vi "Test Sweep API.vi"   [LabVIEW 2019]
uses:
  c3f68086-2c71-4676-baf4-799858c1ae09.vi
  1559a243-b7fb-4211-921b-e5aebecb1ff1.vi
  <vilib>/Analysis/NI_AALBase.lvlib
  <vilib>/Analysis/1siggen.llb/Ramp Pattern by Samples.vi
  cdfe988a-f24c-4ea6-9edf-21cd4fa2a456.vi
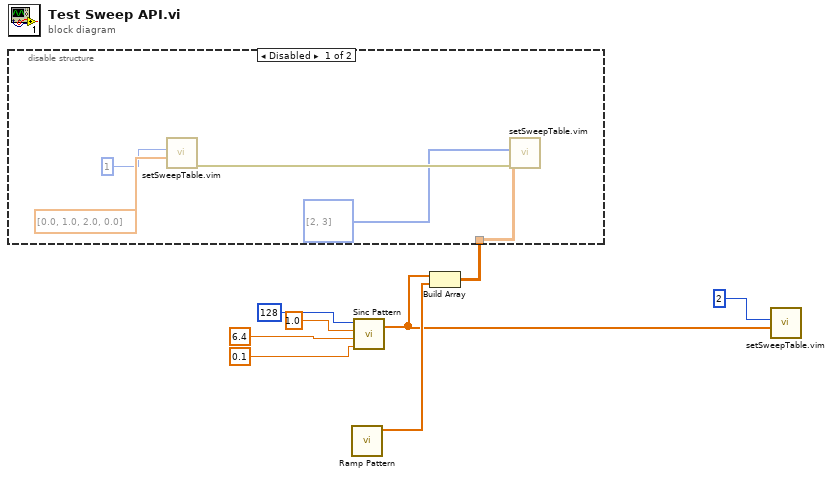
[diagram p0: block diagram]
diagram:
  n1 = call-poly <vilib>:"Ramp Pattern.vi"() -> ("Ramp Pattern"=w7:dbl[])  [unwired: 10 in, 1 out]
  n2 = call <vilib>:"Sinc Pattern.vi"("delta t"=0.1, "delay"=6.4, "amplitude"=1.0, "samples"=128) -> ("Sinc Pattern"=w1:dbl[])  [unwired: 1 out]
  n3 = Build Array(w1, w7) -> (w8:dbl[][])
  n4 = disable-structure shown="Disabled" {
    disable-tunnel: w8 -> [w12 _]
    frame Disabled {
      n5 = call "setSweepTable.vim"("Table"=dbl[] [0.0, 1.0, 2.0, 0.0] ("Pattern"), "Channel"=1) -> ("error out"=w10:errorcluster)  [unwired: 8 in, 1 out]
      n6 = call "setSweepTable.vim"("error in (no error)"=w10, "Table"=w12, "Channel"=i32[] [2, 3] ("Channel 2")) -> ()  [unwired: 7 in, 2 out]
    }
    frame Enabled {
    }
  }
  n7 = call "setSweepTable.vim"("Table"=w1, "Channel"=2) -> ()  [unwired: 8 in, 2 out]
